vi "prac1-3.vi"(2 "Peso Mexicano":dbl) -> (0 "USD":dbl, 1 "EUR":dbl, 4 "JPY":dbl, 5 "GBP":dbl, 6 "CNY":dbl, 7 "RUB":dbl, 8 "INR":dbl, 9 "CAD":dbl, 10 "AUD":dbl)   [LabVIEW 2014]
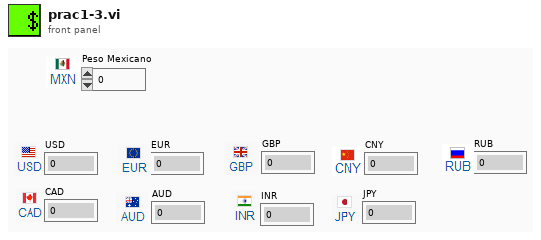
[diagram p1: front panel]
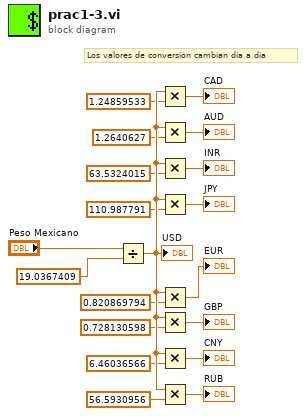
[diagram p0: block diagram]
diagram:
  # "Los valores de conversión cambian día a día"
  n1 = Divide(x="Peso Mexicano", y=19.0367409) -> (x/y=w9:dbl)
  "USD" <- w9
  n2 = Multiply(x=w9, y=1.24859533) -> (x*y=→"CAD":dbl)
  n3 = Multiply(x=w9, y=1.2640627) -> (x*y=→"AUD":dbl)
  n4 = Multiply(x=w9, y=63.5324015) -> (x*y=→"INR":dbl)
  n5 = Multiply(x=w9, y=110.987791) -> (x*y=→"JPY":dbl)
  n6 = Multiply(x=w9, y=0.820869794) -> (x*y=→"EUR":dbl)
  n7 = Multiply(x=w9, y=0.728130598) -> (x*y=→"GBP":dbl)
  n8 = Multiply(x=w9, y=6.46036566) -> (x*y=→"CNY":dbl)
  n9 = Multiply(x=w9, y=56.5930956) -> (x*y=→"RUB":dbl)
